vi "Write Execution Time.vi"(8 "error in":errorcluster, 10 "Values in":dbl[](array[numeric]), 11 "Execution Unit in":refnum<class "Execution Unit.lvclass">) -> (0 "error out":errorcluster, 2 "Values out":dbl[](array[numeric]), 3 "Execution Unit out":refnum<class "Execution Unit.lvclass">)   [LabVIEW 2020, in "AIM ARINC 429 Engine.lvlib" / "Implementation.lvlib" / "Execution Unit.lvclass"]
uses:
  Execution Unit.lvclass
  Execution Unit.lvclass/Execution Unit.ctl
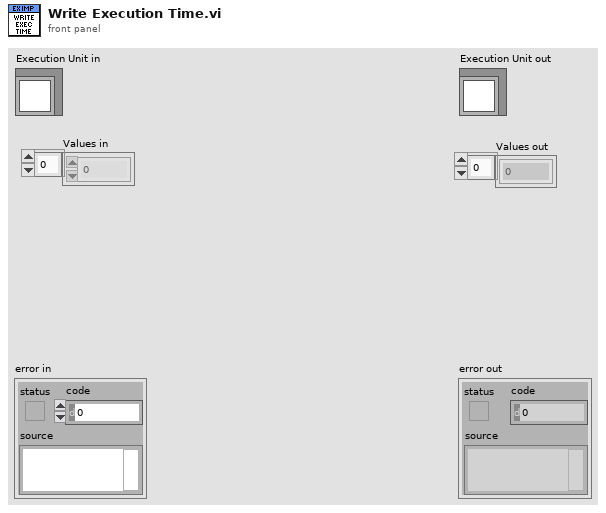
[diagram p1: front panel]
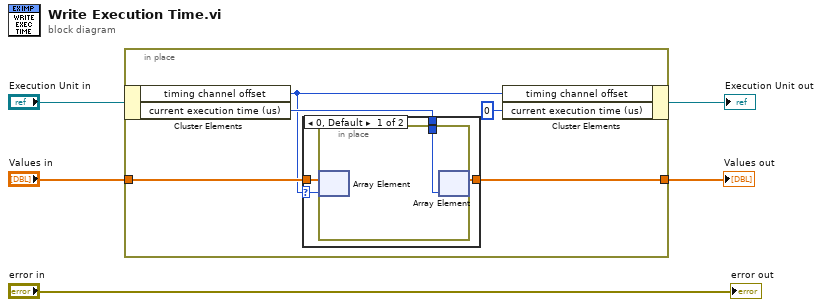
[diagram p0: block diagram]
diagram:
  n1 = in-place {
    in-place-border: "Values in" -> [w10]
    in-place-border: [w9] -> w1
    n2 = in-place-cluster #1("Execution Unit in") -> ("timing channel offset"=w6:i64, "current execution time (us)"=w8:u32)
    n3 = case shown="0, Default" w6 {
      selector: w6 -> [w11 _]
      tunnel: w10 -> [w14 w16]
      tunnel: [w13 w16] -> w9
      tunnel: w8 -> [w12 _]
      frame 0, Default {
        n4 = in-place {
          in-place-border: w12 -> [w15]
          n5 = in-place-array #2(w14, w11) -> ()  [unwired: 1 out]
          n6 = in-place-array #2(w15) -> (w13:dbl[])  [unwired: 1 out]
        }
      }
      frame ..-1 {
      }
    }
    n7 = in-place-cluster #1("timing channel offset"=w6, "current execution time (us)"=u32 0) -> (→"Execution Unit out":refnum<class "Execution Unit.lvclass">)
  }
  "Values out" <- w1
  "error out" <- "error in"
